vi "ExampleQueryServer.vi"() -> ()   [LabVIEW 2019]
uses:
  VIs/labview-grpc-query-server.lvlib
  VIs/gprc-support.lvlib
panel:
  in  "Server Key File (.key)":path
  in  "Server Certificate File (.crt)":path
  in  "stop":bool
  in  "Server Address":string="0.0.0.0:50051"
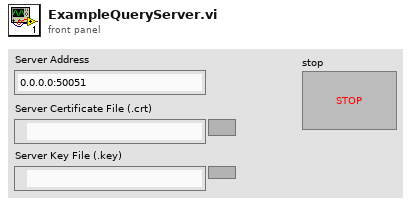
[diagram p1: front panel]
types:
  T1 = typedef "gprc-support.lvlib/grpcId.ctl" = u64
  T2 = cluster{"QueryServer_Invoke":refnum<user-event>, "QueryServer_Query":refnum<user-event>, "QueryServer_Register":refnum<user-event>, "QueryServer_TestDataTypes":refnum<user-event>, "serverId":T1}
  T3 = typedef "labview-grpc-query-server.lvlib/QueryServer_gRPCid.ctl" = u64
  T4 = typedef "labview-grpc-query-server.lvlib/QueryServer_TestDataTypesParameters.ctl" = cluster{"Root":string, "Repeated String":string[], "Repeated Int32":i32[], "Root Int32":i32, "Root Bool":bool, "Repeated Double":dbl[], "Root Double":dbl, "Repeated Bool":bool[], "Root Float":sgl, "Repeated Float":sgl[], "DataTypeTest":T5, "Repeated Nested":T5[]}
  T5 = typedef "labview-grpc-query-server.lvlib/QueryServer_DataTypeTest.ctl" = cluster{"Bool Value":bool, "Int Value":i32, "Float Value":sgl, "Double Value":dbl}
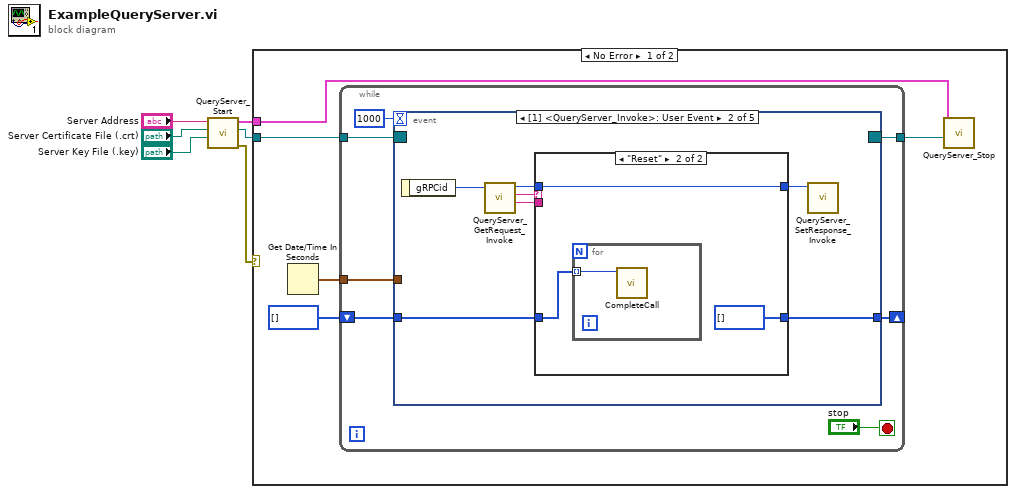
[diagram p0: block diagram]
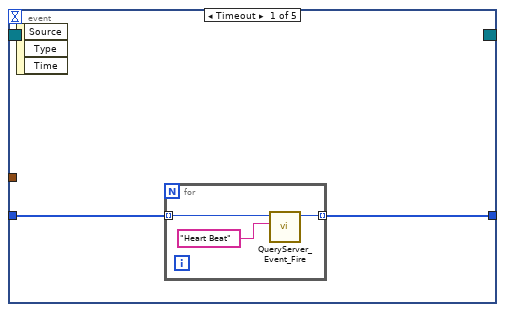
[diagram p2: hidden frame]
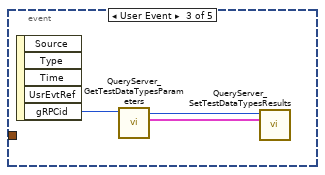
[diagram p4: hidden frame]
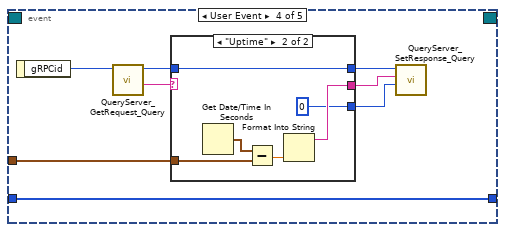
[diagram p5: hidden frame]
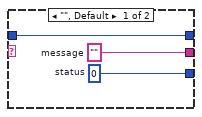
[diagram p6: hidden frame]
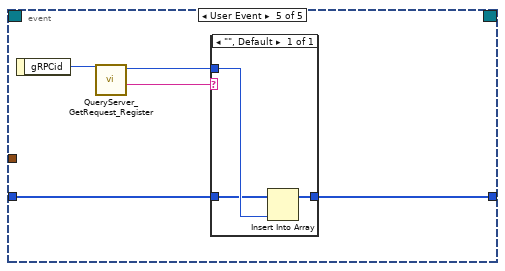
[diagram p7: hidden frame]
diagram:
  n1 = call "QueryServer_Start.vi"("Server Key File (.key)"="Server Key File (.key)", "Server Certificate File (.crt)"="Server Certificate File (.crt)", "Server Address"="Server Address") -> ("error out"=w2:errorcluster, "Event Registration Refnum"=w1:refnum<event-registration>, "Server Info"=w5:T2)  [unwired: 5 in]
  n2 = case shown="No Error" w2 {
    tunnel: w5 -> [w9 _]
    tunnel: w1 -> [w7 _]
    frame No Error {
      n3 = Get Date/Time In Seconds() -> (seconds since 1Jan1904=w11:timestamp)
      n4 = while {
        tunnel: [w17] -> w8
        tunnel: w11 -> [w16]
        shift-right: [w14] -> _
        shift-left: u64[] [] -> [w13]
        tunnel: w7 -> [w12]
        stop <- "stop" stop-if-true
        n5 = event shown="[1] <QueryServer_Invoke>: User Event" {
          selector: w12 -> [_ _ _ _ _]
          dyn-events: [_ _ _ _ _] -> w17
          timeout: 1000 -> [_ _ _ _ _]
          tunnel: w16 -> [_ _ _ w42 _]
          tunnel: [w20 w24 _ w41 w59] -> w14
          tunnel: w13 -> [w19 w25 _ w41 w58]
          event Timeout {
            n6 = event-data() -> ()  [unwired: 1 in, 3 out]
            n7 = for {
              tunnel: w19 -> [w23] mode=indexing
              tunnel: [w21] -> w20 mode=indexing
              n8 = call "QueryServer_Event_Fire.vi"("eventdata"="Heart Beat", "gRPCid"=w23) -> ("gRPCid out"=w21:T1)  [unwired: 8 in, 1 out]
            }
          }
          event User Event {
            n9 = event-data() -> ("gRPCid"=w30:T3)  [unwired: 1 in]
            n10 = call "QueryServer_GetRequest_Invoke.vi"("gRPCid"=w30) -> ("parameter"=w26:string, "command"=w29:string, "gRPCid out"=w28:T1)  [unwired: 5 in, 1 out]
            n11 = case shown="\"Reset\"" w29 {
              tunnel: w28 -> [w32 w33]
              tunnel: [w32 w33] -> w27
              tunnel: w26 -> [_ _]
              tunnel: w25 -> [w31 w35]
              tunnel: [w31 u64[] []] -> w24
              frame "", Default {
              }
              frame "Reset" {
                n12 = for {
                  tunnel: w35 -> [w36] mode=indexing
                  n13 = call "CompleteCall.vi"("gRPCid"=w36) -> ()  [unwired: 9 in, 1 out]
                }
              }
            }
            n14 = call "QueryServer_SetResponse_Invoke.vi"("gRPCid"=w27) -> ()  [unwired: 9 in, 1 out]
          }
          event User Event {
            n15 = event-data() -> ("gRPCid"=w39:T3)  [unwired: 1 in, 4 out]
            n16 = call "QueryServer_GetTestDataTypesParameters.vi"("gRPCid"=w39) -> ("TestDataTypesParameters"=w38:T4, "gRPCid out"=w37:T1)  [unwired: 6 in, 1 out]
            n17 = call "QueryServer_SetTestDataTypesResults.vi"("TestDataTypesParameters"=w38, "gRPCid"=w37) -> ()  [unwired: 6 in, 2 out]
          }
          event User Event {
            n18 = event-data() -> ("gRPCid"=w47:T3)  [unwired: 1 in]
            n19 = call "QueryServer_GetRequest_Query.vi"("gRPCid"=w47) -> ("gRPCid out"=w46:T1, "query"=w40:string)  [unwired: 7 in, 1 out]
            n20 = case shown="\"Uptime\"" w40 {
              tunnel: w46 -> [w50 w52]
              tunnel: [w50 w52] -> w45
              tunnel: [w49 w53] -> w44
              tunnel: [w48 0 ("status")] -> w43
              tunnel: w42 -> [_ w55]
              frame "", Default {
                w48 = 0  # status
                w49 = ""  # message
              }
              frame "Uptime" {
                n21 = Get Date/Time In Seconds() -> (seconds since 1Jan1904=w56:timestamp)
                n22 = Subtract(x=w56, y=w55) -> (x-y=w54:dbl)
                n23 = Format Into String(w54) -> (resulting string=w53:string)  [unwired: 3 in, 1 out]
              }
            }
            n24 = call "QueryServer_SetResponse_Query.vi"("gRPCid"=w45, "message"=w44, "status"=w43) -> ()  [unwired: 7 in, 1 out]
          }
          event User Event {
            n25 = event-data() -> ("gRPCid"=w61:T3)  [unwired: 1 in]
            n26 = call "QueryServer_GetRequest_Register.vi"("gRPCid"=w61) -> ("gRPCid out"=w60:T1, "eventname"=w57:string)  [unwired: 7 in, 1 out]
            n27 = case shown="\"\", Default" w57 {
              tunnel: w60 -> [w64]
              tunnel: [w63] -> w59
              tunnel: w58 -> [w62]
              frame "", Default {
                n28 = Insert Into Array(array=w62, new element=w64) -> (w63:T1[])  [unwired: 1 in]
              }
            }
          }
        }
      }
      n29 = call "QueryServer_Stop.vi"("Server Info"=w9, "Event Registration Refnum"=w8) -> ()  [unwired: 8 in, 1 out]
    }
    frame Error {
    }
  }
